vi "Update Tree Item Description.vi"(11 "UI Data in":refnum<class "Settings UI.lvclass">) -> (3 "UI Data out":refnum<class "Settings UI.lvclass">)   [LabVIEW 2020, in "Output Sequencer.lvlib" / "Settings UI.lvclass"]
uses:
  Settings UI.lvclass
  Settings UI.lvclass/Settings UI.ctl
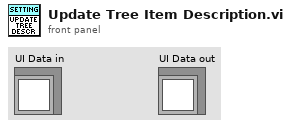
[diagram p1: front panel]
types:
  T1 = typedef "Output Sequencer.lvlib/Settings UI.lvclass/Tree Item Settings.ctl" = cluster{"Tree Label":string, "Indent Level":i32, "Data Type":T2, "Numeric Range":cluster{"Min":dbl, "Max":dbl, "Inc":dbl}, "Allowed Values":string[], "Default Value":string, "Description":string}
  T2 = typedef "Output Sequencer.lvlib/Settings UI.lvclass/Data Type.ctl" = i16
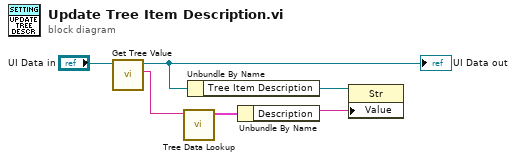
[diagram p0: block diagram]
diagram:
  n1 = call "Get Tree Value.vi"("UI Data in"="UI Data in") -> ("Value"=w1:string, "UI Data out"=w2:refnum<class "Settings UI.lvclass">)  [unwired: 9 in]
  "UI Data out" <- w2
  n2 = call "Tree Data Lookup.vi"("Tag in"=w1) -> ("Tree Data"=w5:T1)  [unwired: 5 in, 5 out]
  n3 = Unbundle By Name(w2) -> ("Tree Item Description"=w4:refnum<vi>)
  n4 = Unbundle By Name(w5) -> ("Description"=w6:string)
  n5 = property class="Str"(reference=w4, "Value"=w6) -> ()  [unwired: 1 in, 2 out]
